vi "Init XY Controller.vi"(6 "Interlock Q Class":refnum<class "Interlock Q Class.lvclass">, 8 "error in (no error)":errorcluster, 9 "Process State Data":refnum<data-value>, 10 "Stage State Data":refnum<data-value>, 11 "XY Stage Controller":refnum<class "XY Stage Controller.lvclass">) -> (0 "error out":errorcluster, 3 "XY Stage Controller":refnum<class "XY Stage Controller.lvclass">)   [LabVIEW 2022 SP3, in "XY Stage Controller.lvclass"]
uses:
  XY Stage Controller.lvclass
  XY Stage Data Class/XY Stage Data Class.lvclass
  Process Framework/Process State Data/Process State Data.lvclass
  Process Framework/Interlock Q Class/Interlock Q Class.lvclass
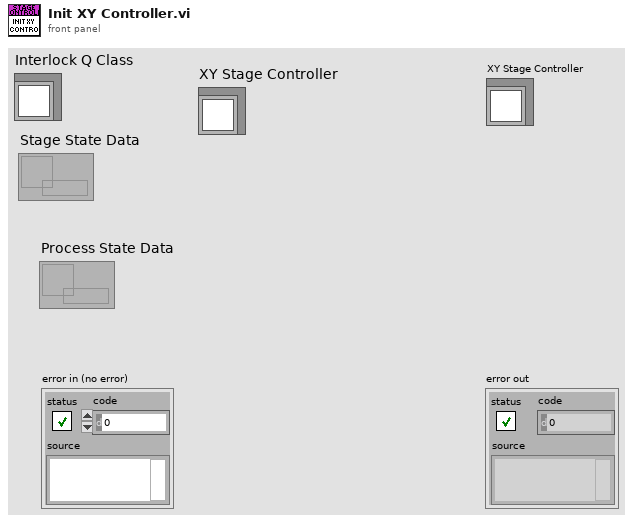
[diagram p1: front panel]
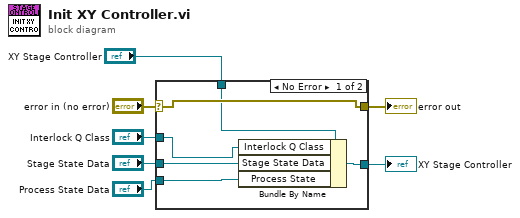
[diagram p0: block diagram]
diagram:
  n1 = case shown="No Error" "error in (no error)" {
    selector: "error in (no error)" -> [w13 w14]
    tunnel: [w13 w14] -> w6
    tunnel: "Interlock Q Class" -> [w9 _]
    tunnel: [w12 _] -> w5
    tunnel: "Stage State Data" -> [w11 _]
    tunnel: "Process State Data" -> [w10 _]
    tunnel: "XY Stage Controller" -> [w8 _]
    frame No Error {
      n2 = Bundle By Name(cluster=w8, "Interlock Q Class"=w9, "Stage State Data"=w11, "Process State"=w10) -> (w12:refnum<class "XY Stage Controller.lvclass">)
    }
    frame Error {
    }
  }
  "error out" <- w6
  "XY Stage Controller" <- w5
